vi "PID.vi"() -> ()   [LabVIEW 2011]
uses:
  <vilib>/addons/control/pid/pid.llb/PID (DBL).vi
  <vilib>/addons/control/pid/NI_PID_pid.lvlib
panel:
  in  "Odometry Data 2":dbl(slide) caption="command heading (rad)" scale=0.0..360.0
  out "speed out":dbl(knob) scale=0.0..10.0
  in  "scale":dbl(knob) scale=0.0..1.0
  out "delta":dbl
  in  "output range":cluster{"output high":dbl, "output low":dbl}={"output high"=100.0, "output low"=-100.0} {"output low" format="%.2f"; "output high" format="%.2f"}
  in  "PID gains":T1={"proportional gain (Kc)"=1.0, "integral time (Ti, min)"=0.01, "derivative time (Td, min)"=0.0}
  out "output":dbl(slide) scale=-10.0..10.0
  in  "Odometry Data":dbl[](array[numeric])
  in  "command heading (rad)":dbl(slide) scale=0.0..360.0
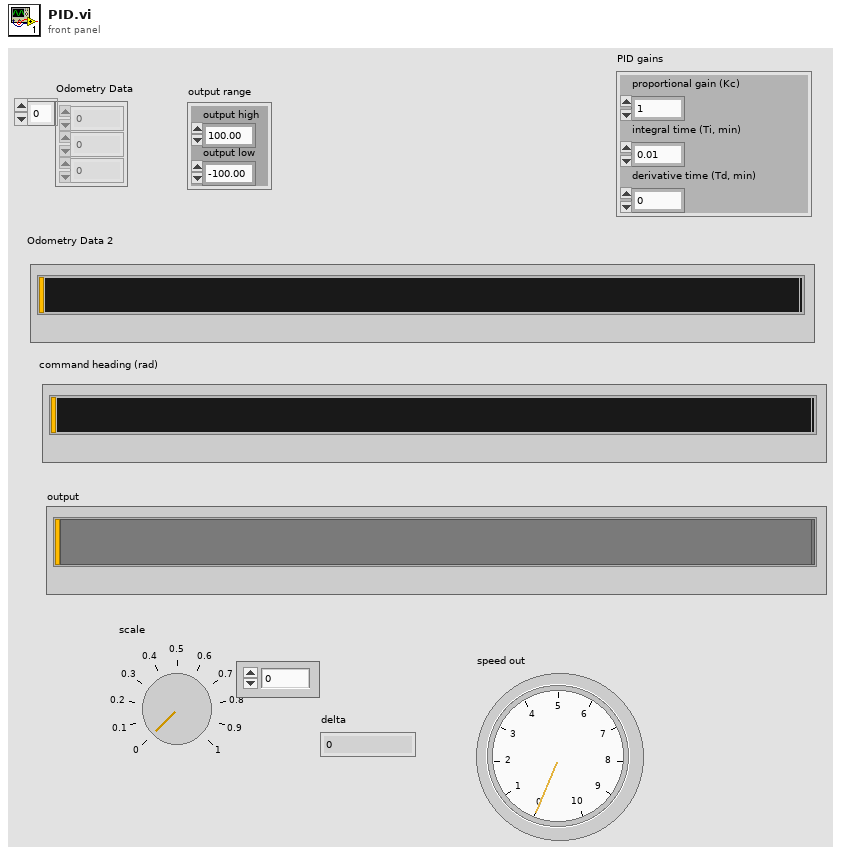
[diagram p1: front panel]
types:
  T1 = cluster{"proportional gain (Kc)":dbl, "integral time (Ti, min)":dbl, "derivative time (Td, min)":dbl}
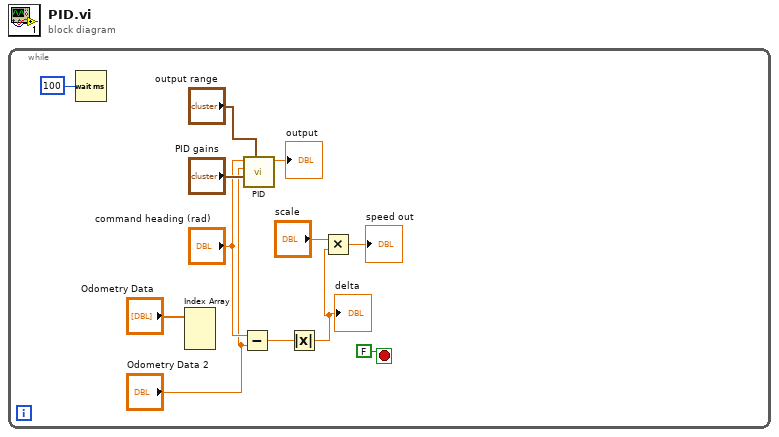
[diagram p0: block diagram]
diagram:
  n1 = while {
    stop <- FALSE stop-if-true
    n2 = Wait (ms)(milliseconds to wait=u32 100) -> ()  [unwired: 1 out]
    n3 = Index Array(array="Odometry Data") -> ()  [unwired: 3 in, 3 out]
    n4 = Subtract(x="command heading (rad)", y="Odometry Data 2") -> (x-y=w6:dbl)
    n5 = call-poly <vilib>:"PID.vi"("output range"="output range", "PID gains"="PID gains", "process variable"="Odometry Data 2", "setpoint"="command heading (rad)") -> ("output"=→"output":dbl)  [unwired: 6 in, 1 out]
    n6 = Absolute Value(x=w6) -> (abs(x)=w4:dbl)
    "delta" <- w4
    n7 = Multiply(x="scale", y=w4) -> (x*y=→"speed out":dbl)
  }
